vi "Main.vi"(8 "error in":errorcluster, 11 "Oscilloscope in":refnum<class "Oscilloscope.lvclass">) -> (0 "error out":errorcluster, 3 "Oscilloscope out":refnum<class "Oscilloscope.lvclass">)   [LabVIEW 2025, in "Oscilloscope.lvclass"]
doc: "The <b>Queued Message Handler</b> of the Worker that owns this VI."
uses:
  Oscilloscope.lvclass
  Oscilloscope.lvclass/Oscilloscope.ctl
  Initialization Data.ctl
  Response Cases.ctl
  rwr_WriteScopeSetup.ctl
  rwr_WriteScopeSetup Reply.ctl
  rqp_ReadScopeWaveform.ctl
  <vilib>/addons/_Workers/Library/Case Label.ctl
  <vilib>/addons/_Workers/Library/Workers.lvlib
  rsp_WaveformDataRuturn.ctl
panel:
  out "SetupType":string
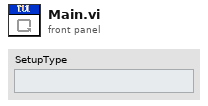
[diagram p1: front panel]
types:
  T1 = typedef "Oscilloscope.lvclass/Initialization Data.ctl" = cluster{"Response Cases":T2}
  T2 = typedef "Oscilloscope.lvclass/Response Cases.ctl" = cluster{"Placeholder - Can be deleted":string, "WaveformDataRuturn":T3}
  T3 = typedef "Workers.lvlib/Case Label.ctl" = string
  T4 = typedef "Oscilloscope.lvclass/rwr_WriteScopeSetup Reply.ctl" = cluster{"String":string}
  T5 = typedef "Oscilloscope.lvclass/rwr_WriteScopeSetup.ctl" = cluster{"String":string}
  T6 = typedef "Oscilloscope.lvclass/rsp_WaveformDataRuturn.ctl" = cluster{"String":string, "Waveform":waveform(dbl)}
  T7 = typedef "Oscilloscope.lvclass/rqp_ReadScopeWaveform.ctl" = cluster{"String":string}
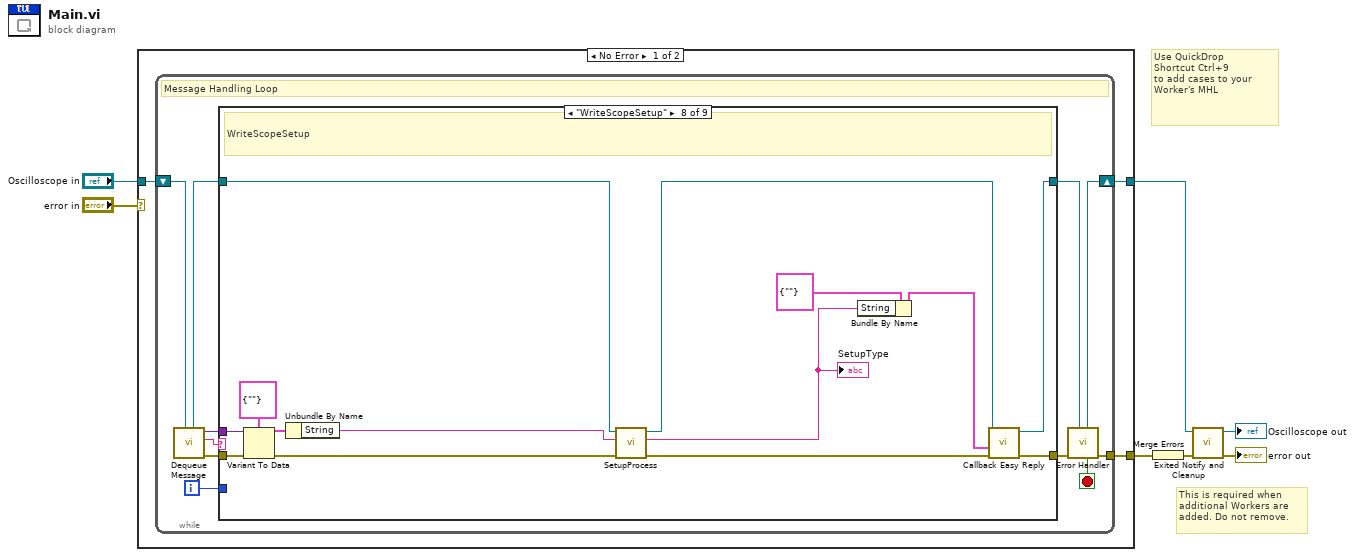
[diagram p0: block diagram]
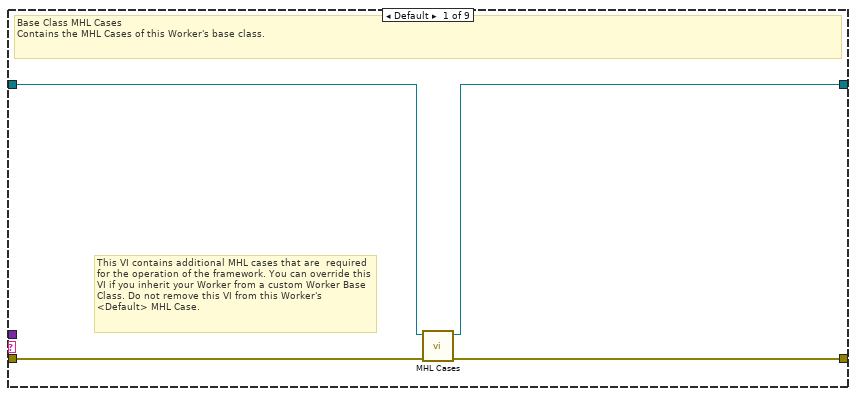
[diagram p2: hidden frame]
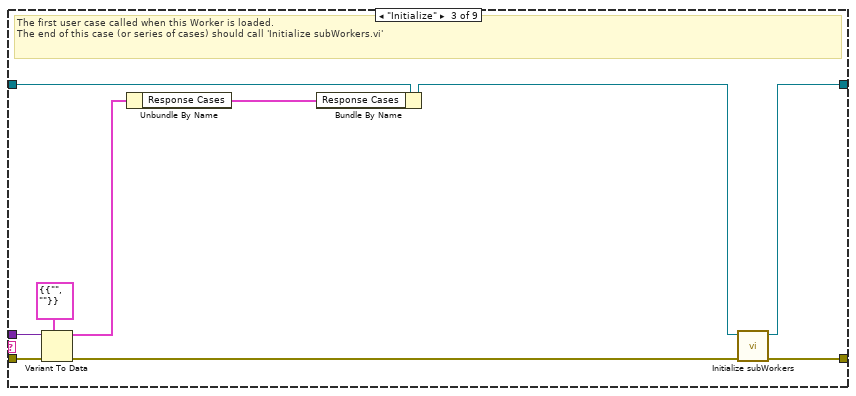
[diagram p4: hidden frame]
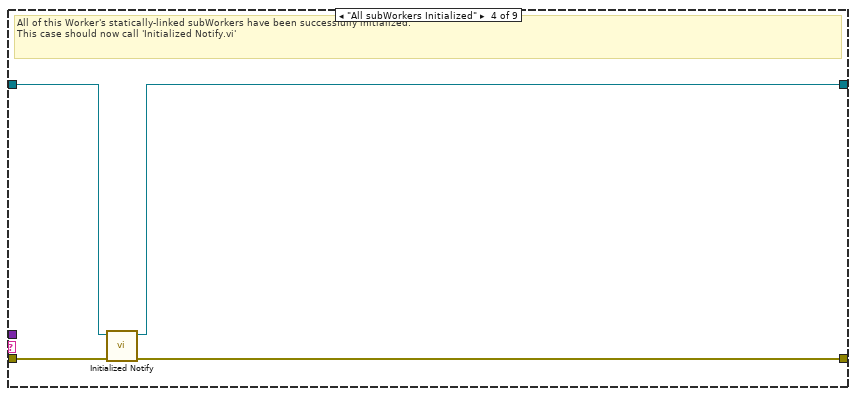
[diagram p5: hidden frame]
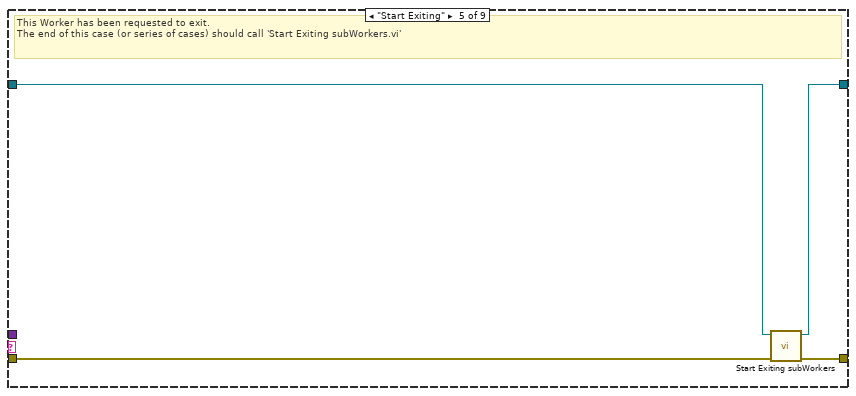
[diagram p6: hidden frame]
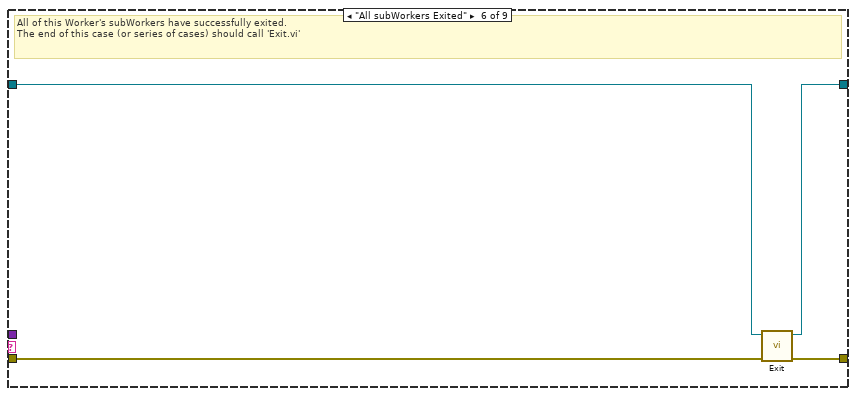
[diagram p7: hidden frame]
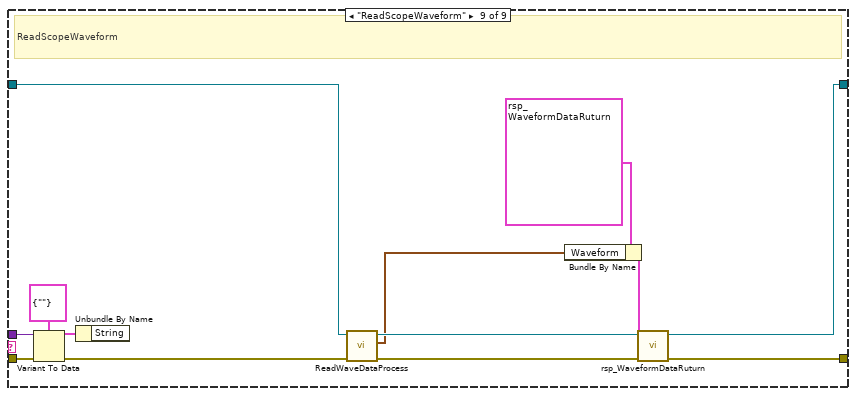
[diagram p9: hidden frame]
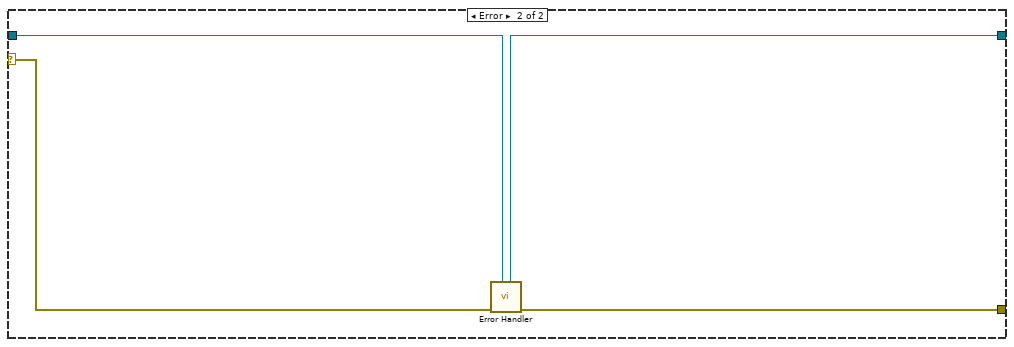
[diagram p10: hidden frame]
diagram:
  # "Use QuickDrop\nShortcut Ctrl+9\nto add cases to your\nWorker's MHL"
  # "This is required when additional Workers are added. Do not remove."
  n1 = case shown="No Error" "error in" {
    tunnel: "Oscilloscope in" -> [w8 w80]
    tunnel: [w10 w81] -> w6
    tunnel: [w9 w79] -> w7
    selector: "error in" -> [_ w82]
    frame No Error {
      n2 = while {
        shift-right: [w19] -> w9
        shift-left: w8 -> [w21]
        tunnel: [w20] -> w10
        i -> [w12]
        stop <- w13 stop-if-true
        # "Message Handling Loop"
        n3 = call-dynamic "Dequeue Message.vi"("Worker"=w21) -> ("error out"=w18:errorcluster, "Case out"=w14:string, "Data out"=w11:variant, "Worker out"=w16:refnum<class "Oscilloscope.lvclass">)  [unwired: 6 in, 1 out]
        n4 = case "Worker MHL Case Structure (DO NOT CHANGE LABEL NAME)" shown="\"WriteScopeSetup\"" w14 {
          tunnel: w18 -> [w25 w26 w35 w41 w42 w49 w51 w65 w78]
          tunnel: [w24 w26 w37 w40 w45 w48 w51 w60 w71] -> w17
          tunnel: w16 -> [w23 w27 w34 w39 w43 w47 w50 w55 w72]
          tunnel: [w22 w27 w36 w38 w44 w46 w50 w59 w69] -> w15
          tunnel: w12 -> [_ _ _ _ _ _ _ _ _]
          tunnel: w11 -> [_ _ w32 _ _ _ _ w62 w75]
          frame Default {
            # "This VI contains additional MHL cases that are  required for the operation of the framework. You can override this VI if you inherit your Worker from a custom Worker Base Class. Do not remove this VI from this Worker's <Default> MHL Case."
            # "Base Class MHL Cases\nContains the MHL Cases of this Worker's base class."
            n5 = call-dynamic "MHL Cases.vi"("error in"=w25, "Worker in"=w23) -> ("error out"=w24:errorcluster, "Worker out"=w22:refnum<class "Oscilloscope.lvclass">)  [unwired: 8 in]
          }
          frame "------------ FRAMEWORK CASES -----------" {
            # "Start of Workers Framework Cases"
          }
          frame "Initialize" {
            # "The first user case called when this Worker is loaded.\nThe end of this case (or series of cases) should call 'Initialize subWorkers.vi'"
            n6 = Variant To Data(error in=w35, type=T1 {"Response Cases"={"Placeholder - Can be deleted"="", "WaveformDataRuturn"=""}} ("Cluster"), Variant=w32) -> (data=w30:T1, error out=w33:errorcluster)
            n7 = Unbundle By Name(w30) -> ("Response Cases"=w29:T2)
            n8 = Bundle By Name(cluster=w34, "Response Cases"=w29) -> (w31:refnum<class "Oscilloscope.lvclass">)
            n9 = call-dynamic "Initialize subWorkers.vi"("error in"=w33, "Worker"=w31) -> ("error out"=w37:errorcluster, "dup Worker out"=w36:refnum<class "Oscilloscope.lvclass">)  [unwired: 8 in]
          }
          frame "All subWorkers Initialized" {
            # "All of this Worker's statically-linked subWorkers have been successfully initialized.\nThis case should now call 'Initialized Notify.vi'"
            n10 = call-dynamic "Initialized Notify.vi"("error in"=w41, "Worker"=w39) -> ("error out"=w40:errorcluster, "dup Worker out"=w38:refnum<class "Oscilloscope.lvclass">)  [unwired: 8 in]
          }
          frame "Start Exiting" {
            # "This Worker has been requested to exit. \nThe end of this case (or series of cases) should call 'Start Exiting subWorkers.vi'"
            n11 = call-dynamic "Start Exiting subWorkers.vi"("error_in"=w42, "Worker"=w43) -> ("error out"=w45:errorcluster, "dup Worker out"=w44:refnum<class "Oscilloscope.lvclass">)  [unwired: 8 in]
          }
          frame "All subWorkers Exited" {
            # "All of this Worker's subWorkers have successfully exited. \nThe end of this case (or series of cases) should call 'Exit.vi'"
            n12 = call-dynamic "Exit.vi"("error_in"=w49, "Worker"=w47) -> ("error out"=w48:errorcluster, "dup Worker out"=w46:refnum<class "Oscilloscope.lvclass">)  [unwired: 8 in]
          }
          frame "------------- PUBLIC API CASES -------------" {
            # "Start of Workers Public API Cases"
          }
          frame "WriteScopeSetup" {
            # "WriteScopeSetup"
            n13 = Variant To Data(error in=w65, type=T5 {"String"=""} ("Data"), Variant=w62) -> (data=w61:T5, error out=w64:errorcluster)
            n14 = Unbundle By Name(w61) -> ("String"=w53:string)
            n15 = call-dynamic "SetupProcess.vi"("error in (no error)"=w64, "SetupData"=w53, "Oscilloscope in"=w55) -> ("error out"=w57:errorcluster, "Type"=w52:string, "Oscilloscope out"=w56:refnum<class "Oscilloscope.lvclass">)  [unwired: 6 in]
            "SetupType" <- w52
            n16 = Bundle By Name(cluster=T4 {"String"=""} ("Reply Data"), "String"=w52) -> (w54:T4)
            n17 = call-dynamic "Callback Easy Reply.vi"("error in"=w57, "Data"=w54, "Worker"=w56) -> ("error out"=w60:errorcluster, "dup Worker out"=w59:refnum<class "Oscilloscope.lvclass">)  [unwired: 7 in]
          }
          frame "ReadScopeWaveform" {
            # "ReadScopeWaveform"
            n18 = Variant To Data(error in=w78, type=T7 {"String"=""} ("Data"), Variant=w75) -> (data=w74:T7, error out=w77:errorcluster)
            n19 = Unbundle By Name(w74) -> ()  [unwired: 1 out]
            n20 = call-dynamic "ReadWaveDataProcess.vi"("error in (no error)"=w77, "Oscilloscope in"=w72) -> ("error out"=w73:errorcluster, "Waveform"=w66:waveform(dbl), "Oscilloscope out"=w70:refnum<class "Oscilloscope.lvclass">)  [unwired: 7 in]
            n21 = Bundle By Name(cluster=T6 {"String"="", "Waveform"={"t0"=timestamp(0 s since 1904-01-01), "dt"=1.0, "Y"=[]}} ("Data in"), "Waveform"=w66) -> (w67:T6)
            n22 = call "rsp_WaveformDataRuturn.vi"("error in"=w73, "Data in"=w67, "Oscilloscope in"=w70) -> ("error out"=w71:errorcluster, "dup Oscilloscope out"=w69:refnum<class "Oscilloscope.lvclass">)  [unwired: 7 in]
          }
        }
        n23 = call-dynamic "Error Handler.vi"("Worker"=w15, "error_in"=w17) -> ("error out"=w20:errorcluster, "Stop Loop"=w13:bool, "Worker out"=w19:refnum<class "Oscilloscope.lvclass">)  [unwired: 7 in]
      }
    }
    frame Error {
      n24 = call-dynamic "Error Handler.vi"("Worker"=w80, "error_in"=w82) -> ("error out"=w81:errorcluster, "Worker out"=w79:refnum<class "Oscilloscope.lvclass">)  [unwired: 7 in, 1 out]
    }
  }
  n25 = Merge Errors(w6) -> (w3:errorcluster)
  n26 = call-dynamic "Exited Notify and Cleanup.vi"("error_in"=w3, "Worker"=w7) -> ("error out"=→"error out":errorcluster, "dup Worker out"=→"Oscilloscope out":refnum<class "Oscilloscope.lvclass">)  [unwired: 8 in]
